vi "Arbitor_Var.vi"(1 "Selector Array":bool[](array[boolean]), 2 "Input Array":variant[](array[variant])) -> (0 "Arbitrated Output":variant)   [LabVIEW 2016]
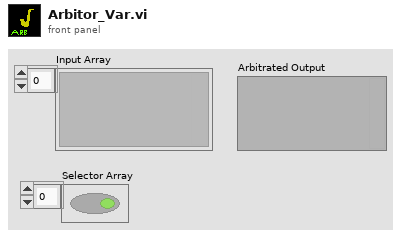
[diagram p1: front panel]
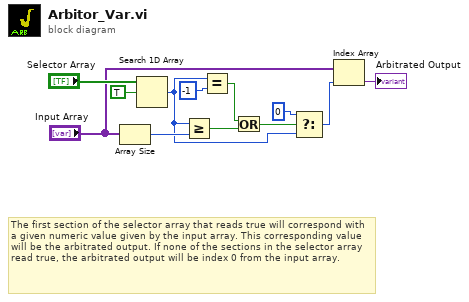
[diagram p0: block diagram]
diagram:
  # "The first section of the selector array that reads true will correspond with a given numeric value given by the input array. This corresponding value will be the arbitrated output. If none of the sections in the selector array read true, the arbitrated output will be index 0 from the input array."
  n1 = Array Size(array="Input Array") -> (size(s)=w7:i32)
  n2 = Search 1D Array(1D array="Selector Array", element=TRUE) -> (index of element=w2:i32)  [unwired: 1 in]
  n3 = Greater Or Equal?(x=w2, y=w7) -> (x >= y?=w6:bool)
  n4 = Equal?(x=w2, y=-1) -> (x = y?=w5:bool)
  n5 = Or(x=w5, y=w6) -> (x .or. y?=w4:bool)
  n6 = Select(t=0, s=w4, f=w2) -> (s? t:f=w1:i32)
  n7 = Index Array(array="Input Array", index=w1) -> (element=→"Arbitrated Output":variant)
